vi "ex_1_FGV.vi"(6 "dx (0,1)":dbl=0.1, 7 "Sinus Action  (Increment argument)":T1=enum."Increment argument", 8 "error in (no error)":errorcluster) -> (0 "error out":errorcluster, 3 "Sinus output":dbl(graph))   [LabVIEW 2020]
uses:
  #typedef_FGV_SinusAction.ctl
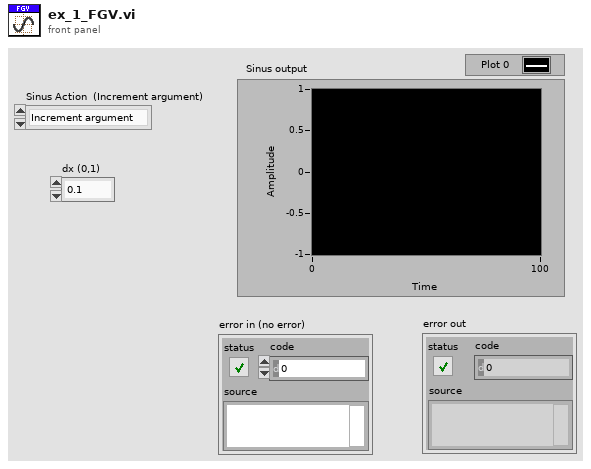
[diagram p1: front panel]
types:
  T1 = typedef "#typedef_FGV_SinusAction.ctl" = enum16{"Reset", "Increment argument"}
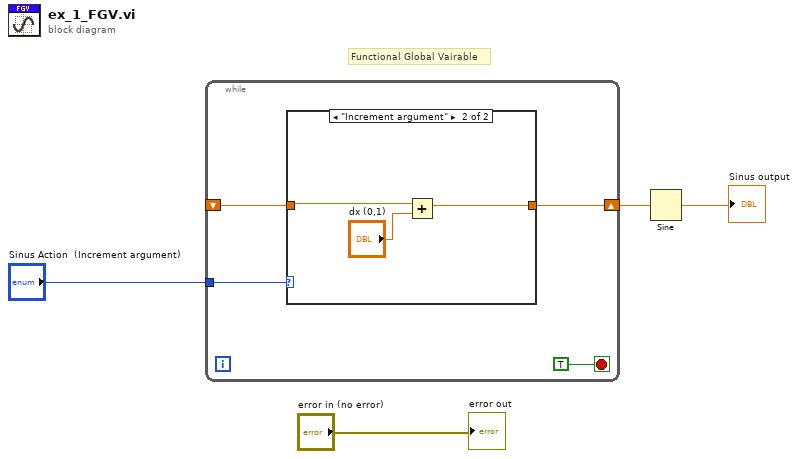
[diagram p0: block diagram]
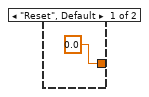
[diagram p2: hidden frame]
diagram:
  # "Functional Global Vairable"
  n1 = while {
    tunnel: "Sinus Action  (Increment argument)" -> [w8]
    shift-right: [w5] -> w2
    shift-left: _ -> [w6]
    stop <- TRUE stop-if-true
    n2 = case shown="\"Increment argument\"" w8 {
      tunnel: w6 -> [_ w10]
      tunnel: [0.0 w11] -> w5
      frame "Reset", Default {
      }
      frame "Increment argument" {
        n3 = Add(x=w10, y="dx (0,1)") -> (x+y=w11:dbl)
      }
    }
  }
  n4 = Sine(x=w2) -> (sin(x)=→"Sinus output":dbl)
  "error out" <- "error in (no error)"
